vi "Measure.vi"(8 "error in (no error)":errorcluster, 9 "measurement configuration":variant, 10 "measure call context in":refnum<class "Measure Call Context.lvclass">, 11 "measurement plugin in":refnum<class "NI Switch Control.lvclass">) -> (0 "error out":errorcluster, 1 "measurement results":variant, 2 "measure call context out":refnum<class "Measure Call Context.lvclass">, 3 "measurement plugin out":refnum<class "NI Switch Control.lvclass">)   [LabVIEW 2025, in "NI Switch Control.lvclass"]
uses:
  NI Switch Control.lvclass
  <vilib>/Plug-In SDKs/Measurements/Measure Call Context/Measure Call Context.lvclass
  Measurement Configuration.ctl
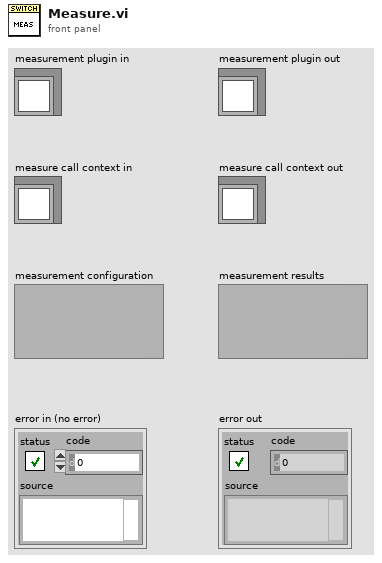
[diagram p1: front panel]
types:
  T1 = typedef "NI Switch Control.lvclass/Measurement Configuration.ctl" = cluster{"TREE":string, "CONNECTIONS":i32, "START":bool, "OPEN SESSION":bool, "OPERATION":i32, "SWITCH EXECUTIVE VIRTUAL DEVICE":string}
  T2 = typedef "NI Switch Control.lvclass/Measurement Results.ctl" = cluster{"START":bool, "OPEN SESSION":bool, "SWITCH EXECUTIVE VIRTUAL DEVICE":string, "TREE":string, "CONNECTIONS":i32, "OPERATION":i32}
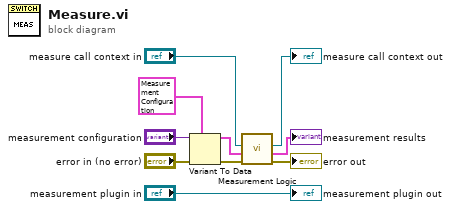
[diagram p0: block diagram]
diagram:
  n1 = Variant To Data(error in="error in (no error)", type=T1 {"TREE"="Lorem ipsum dolor sit", "CONNECTIONS"=1, "START"=TRUE, "OPEN SESSION"=FALSE, "OPERATION"=32, "SWITCH EXECUTIVE VIRTUAL DEVICE"="Empty"} ("measurement configuration"), Variant="measurement configuration") -> (data=w1:T1, error out=w7:errorcluster)
  n2 = call "Measurement Logic.vi"("error in"=w7, "measurement configuration"=w1, "measure call context in"="measure call context in") -> ("error out"=→"error out":errorcluster, "measurement results"=→"measurement results":T2, "measure call context out"=→"measure call context out":refnum<class "Measure Call Context.lvclass">)  [unwired: 6 in]
  "measurement plugin out" <- "measurement plugin in"
